vi "Integrate Encoders (SubVI).vi"(10 "dt":dbl, 11 "NI_Robotics_Steering Frame in":T1) -> (3 "Estimated Pose Delta":cluster{dbl, dbl, dbl})   [LabVIEW 2017]
uses:
  <vilib>/robotics/Steering/Class Type Definitions/Steering Frame.ctl
  <vilib>/robotics/Steering/Steering Frame/NI_Robotics_Steering Frame.lvclass
  <vilib>/robotics/Steering/Steering Frame/Get Steering Frame Velocity from Motors.vi
  <vilib>/robotics/Steering/Class Type Definitions/NI_Robotics_Steering Class Types.lvlib
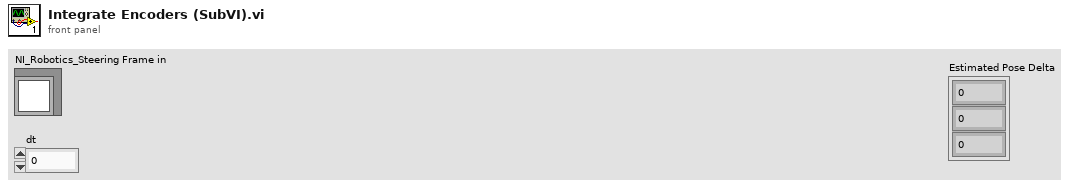
[diagram p1: front panel]
types:
  T1 = typedef "NI_Robotics_Steering Class Types.lvlib/Steering Frame.ctl" = refnum<class "NI_Robotics_Steering Frame.lvclass">
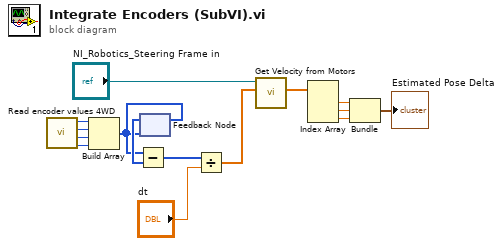
[diagram p0: block diagram]
diagram:
  n1 = call "Read encoder values 4WD.vi"() -> ("Back right"=w10:i32, "Back left"=w9:i32, "Front right"=w8:i32, "Front left"=w7:i32)  [unwired: 8 in]
  n2 = Build Array(w7, w8, w9, w10) -> (w1:i32[])
  n3 = feedback #1(w1) -> (w15:i32[])
  n4 = Subtract(x=w1, y=w15) -> (x-y=w12:i32[])
  n5 = feedback-in #1(w1) -> ()
  n6 = Divide(x=w12, y="dt") -> (x/y=w13:dbl[])
  n7 = call-poly <vilib>:"Get Velocity from Motors.vi"("ccw motor velocity states"=w13, "steering frame in"="NI_Robotics_Steering Frame in") -> ("estimated steering frame velocity"=w6:dbl[])  [unwired: 7 in, 2 out]
  n8 = Index Array(array=w6) -> (element #1=w5:dbl, element #2=w4:dbl, element #3=w3:dbl)  [unwired: 3 in]
  n9 = Bundle(w5, w4, w3) -> (→"Estimated Pose Delta":cluster{dbl, dbl, dbl})  [unwired: 1 in]
